vi "coil polarity pattern reader.vi"(11 "polarity pattern file":path) -> (0 "numSweeps list":i64[](array[numeric]), 3 "polarity list":i64[](array[numeric]))   [LabVIEW 2020]
uses:
  <vilib>/Utility/file.llb/Read Delimited Spreadsheet (I64).vi
panel:
  out "full sweep pattern":i64[][](array[numeric])
  # "0 means - current\n1 means + current"
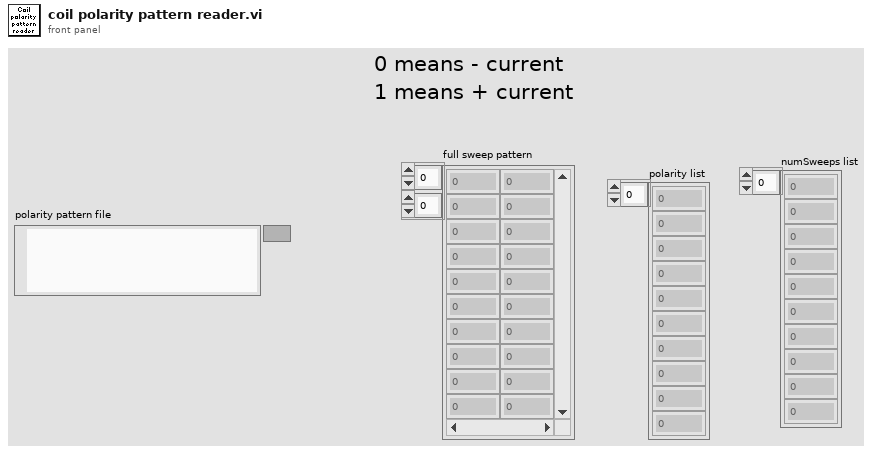
[diagram p1: front panel]
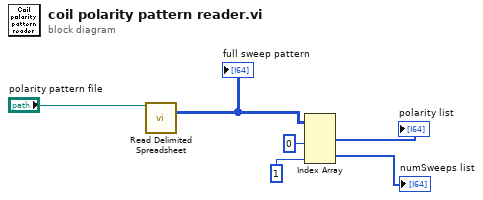
[diagram p0: block diagram]
diagram:
  n1 = call-poly <vilib>:"Read Delimited Spreadsheet.vi"("file path (dialog if empty)"="polarity pattern file") -> ("all rows"=w5:i64[][])  [unwired: 9 in, 5 out]
  "full sweep pattern" <- w5
  n2 = Index Array(array=w5, index (col) #1=0 ("disabled index (col)"), index (col) #2=1 ("disabled index (col)")) -> (element #1=→"polarity list":i64[], element #2=→"numSweeps list":i64[])  [unwired: 2 in]
